vi "Read Channels to scan.vi"(8 "error in (no error)":errorcluster, 11 "Instrument with scanner.lvclass in":refnum<class "Instrument with scanner.lvclass">) -> (0 "error out":errorcluster, 1 "Seconds between samples":dbl=1.0 format="%_4f", 2 "Channels to scan (empty - don't use scanner option)":i32[](array[numeric]), 3 "Instrument with scanner.lvclass out":refnum<class "Instrument with scanner.lvclass">)   [LabVIEW 2015, in "Instrument with scanner.lvclass"]
uses:
  Instrument with scanner.lvclass
  Instrument with scanner.lvclass/Instrument with scanner.ctl
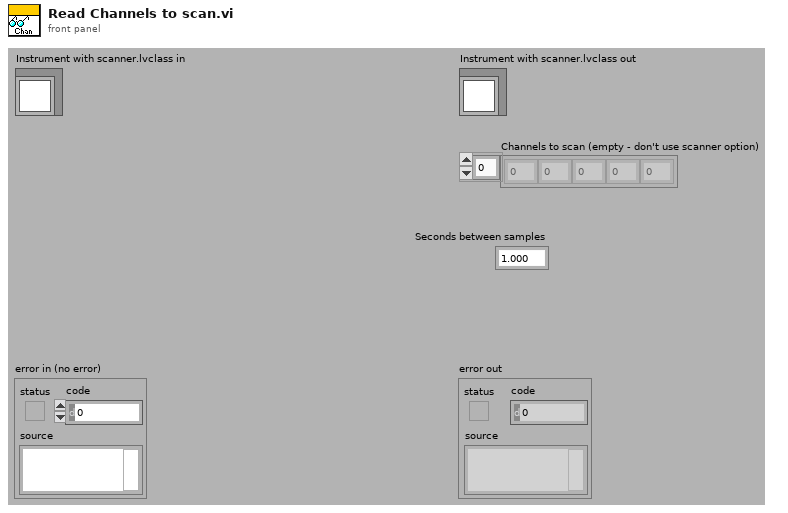
[diagram p1: front panel]
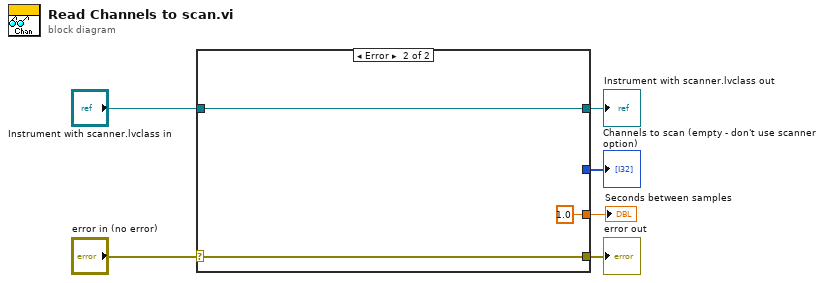
[diagram p0: block diagram]
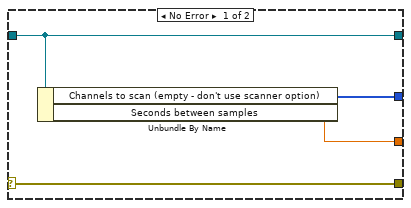
[diagram p2: hidden frame]
diagram:
  n1 = case shown="Error" "error in (no error)" {
    selector: "error in (no error)" -> [w10 w12]
    tunnel: [w10 w12] -> w5
    tunnel: [w9 w13] -> w3
    tunnel: "Instrument with scanner.lvclass in" -> [w9 w13]
    tunnel: [w8 _] -> w2
    tunnel: [w7 1.0 ("Seconds between samples")] -> w1
    frame No Error {
      n2 = Unbundle By Name(w9) -> ("Channels to scan (empty - don't use scanner option)"=w8:i32[], "Seconds between samples"=w7:dbl)
    }
    frame Error {
    }
  }
  "error out" <- w5
  "Instrument with scanner.lvclass out" <- w3
  "Channels to scan (empty - don't use scanner option)" <- w2
  "Seconds between samples" <- w1
